vi "OCR Get Names.vi"(7 "error in":errorcluster, 10 "SS Path":path=path "c:/PokerSS/SS.png") -> (0 "error out":errorcluster, 3 "Player Names":string[](array[string]))   [LabVIEW 2015]
uses:
  <vilib>/vision/NI_Vision_Development_Module.lvlib
panel:
  out "Image Out":T1(plugin-control)
  out "String ( Player10 OCR/OCV 4)":string
  out "String (Player9 OCR/OCV 4)":string
  out "String (Player8 OCR/OCV 4)":string
  out "String (Player7 OCR/OCV 4)":string
  out "String (Playe6 OCR/OCV 4)":string
  out "String (Player5 OCR/OCV 4)":string
  out "String (Player4 OCR/OCV 4)":string
  out "String (Player3 OCR/OCV 4)":string
  out "String (Player2 OCR/OCV 4)":string
  out "String (Player1 OCR/OCV 4)":string
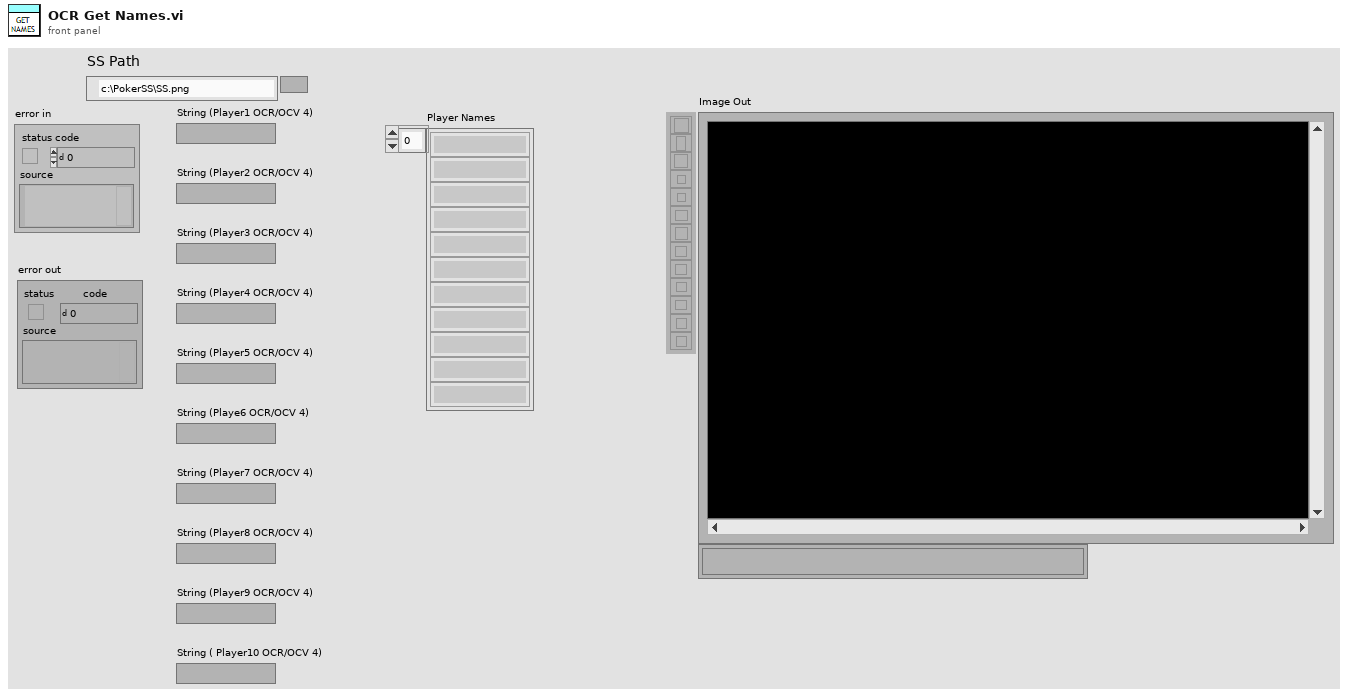
[diagram p1: front panel]
types:
  T1 = typedef "IMAQ Image.ctl" = refnum<image>
  T2 = cluster{"Threshold Data":cluster{"Method":enum16{"Fixed Range", "Uniform", "Linear", "Non Linear", "Local", "Color"}, "Looking for":u32, "Color Mode":u32, "Kernel Size":cluster{"Width":i32, "Height":i32}, "Ranges":cluster{"Min":i32, "Max":i32}[]}, "Reject Border":bool, "Number Of Erosions":i32, "Size & Spacing":cluster{"Segment Algorithm":u16, "Min Bounding Rect Width":i32, "Max Bounding Rect Width":i32, "Min Bounding Rect Height":i32, "Max Bounding Rect Height":i32, "Min Character Size":i32, "Max Character Size":i32, "Min Char Spacing":i32, "Max Horiz Element Spacing":i32, "Max Vert Element Spacing":i32, "Max Space Distance":i32}, "Read Options":cluster{"Read Strategy":i32, "Read Resolution":i32, "Scale Dependant":bool, "Aspect Ratio":i32, "Acceptance Level":i32, "Substitution Character":string, "MultiLine":bool}, "Valid Characters":cluster{"Pre-defined characters":i32, "User-defined characters":string}[], "Use Text Pattern":bool, "Orientation":u32, "# Lines Expected":u32, "Number of Blocks":i32}
  T3 = cluster{"Global Rectangle":i32[], "Contours":cluster{"ID":enum32{"External", "Internal"}, "Type":u32, "Coordinates":i32[]}[]}
  T4 = typedef "Image Type" = u32
  T5 = typedef "IMAQ OCR Session.ctl" = refnum<k1>
diagram:
  w25 = u32 0 items=["Grayscale", "Binary", "Gradient", "Rainbow", "Temperature", "User Defined", "Binary 16 Bit", "Gradient 16 Bit", "Rainbow 16 Bit", "Temperature 16 Bit", "User Defined 16 Bit"] ("Palette Type")
  w34 = T2 {"Threshold Data"={"Method"=enum."Linear", "Looking for"=1, "Color Mode"=0, "Kernel Size"={"Width"=32, "Height"=32}, "Ranges"=[{"Min"=1, "Max"=255}]}, "Reject Border"=TRUE, "Number Of Erosions"=0, "Size & Spacing"={"Segment Algorithm"=0, "Min Bounding Rect Width"=2, "Max Bounding Rect Width"=7, "Min Bounding Rect Height"=2, "Max Bounding Rect Height"=65536, "Min Character Size"=4, "Max Character Size"=5555, "Min Char Spacing"=1, "Max Horiz Element Spacing"=1, "Max Vert Element Spacing"=0, "Max Space Distance"=65536}, "Read Options"={"Read Strategy"=1, "Read Resolution"=2, "Scale Dependant"=FALSE, "Aspect Ratio"=400, "Acceptance Level"=700, "Substitution Character"="?", "MultiLine"=FALSE}, "Valid Characters"=[], "Use Text Pattern"=FALSE, "Orientation"=0, "# Lines Expected"=0, "Number of Blocks"=4}  # Parameters
  w35 = T3 {"Global Rectangle"=[718, 479, 831, 496], "Contours"=[{"ID"=enum."External", "Type"=3, "Coordinates"=[718, 479, 831, 496]}]}  # ROI Descriptor
  w43 = T2 {"Threshold Data"={"Method"=enum."Linear", "Looking for"=1, "Color Mode"=0, "Kernel Size"={"Width"=32, "Height"=32}, "Ranges"=[{"Min"=1, "Max"=255}]}, "Reject Border"=TRUE, "Number Of Erosions"=0, "Size & Spacing"={"Segment Algorithm"=0, "Min Bounding Rect Width"=2, "Max Bounding Rect Width"=7, "Min Bounding Rect Height"=2, "Max Bounding Rect Height"=65536, "Min Character Size"=4, "Max Character Size"=5555, "Min Char Spacing"=1, "Max Horiz Element Spacing"=1, "Max Vert Element Spacing"=0, "Max Space Distance"=65536}, "Read Options"={"Read Strategy"=1, "Read Resolution"=2, "Scale Dependant"=FALSE, "Aspect Ratio"=400, "Acceptance Level"=700, "Substitution Character"="?", "MultiLine"=FALSE}, "Valid Characters"=[], "Use Text Pattern"=FALSE, "Orientation"=0, "# Lines Expected"=0, "Number of Blocks"=4}  # Parameters
  w44 = T3 {"Global Rectangle"=[523, 517, 648, 536], "Contours"=[{"ID"=enum."External", "Type"=3, "Coordinates"=[523, 517, 648, 536]}]}  # ROI Descriptor
  w52 = T2 {"Threshold Data"={"Method"=enum."Linear", "Looking for"=1, "Color Mode"=0, "Kernel Size"={"Width"=32, "Height"=32}, "Ranges"=[{"Min"=1, "Max"=255}]}, "Reject Border"=TRUE, "Number Of Erosions"=0, "Size & Spacing"={"Segment Algorithm"=0, "Min Bounding Rect Width"=2, "Max Bounding Rect Width"=7, "Min Bounding Rect Height"=2, "Max Bounding Rect Height"=65536, "Min Character Size"=4, "Max Character Size"=5555, "Min Char Spacing"=1, "Max Horiz Element Spacing"=1, "Max Vert Element Spacing"=0, "Max Space Distance"=65536}, "Read Options"={"Read Strategy"=1, "Read Resolution"=2, "Scale Dependant"=FALSE, "Aspect Ratio"=400, "Acceptance Level"=700, "Substitution Character"="?", "MultiLine"=FALSE}, "Valid Characters"=[], "Use Text Pattern"=FALSE, "Orientation"=0, "# Lines Expected"=0, "Number of Blocks"=4}  # Parameters
  w53 = T3 {"Global Rectangle"=[389, 674, 500, 690], "Contours"=[{"ID"=enum."External", "Type"=3, "Coordinates"=[389, 674, 500, 690]}]}  # ROI Descriptor
  w61 = T2 {"Threshold Data"={"Method"=enum."Linear", "Looking for"=1, "Color Mode"=0, "Kernel Size"={"Width"=32, "Height"=32}, "Ranges"=[{"Min"=1, "Max"=255}]}, "Reject Border"=TRUE, "Number Of Erosions"=0, "Size & Spacing"={"Segment Algorithm"=0, "Min Bounding Rect Width"=2, "Max Bounding Rect Width"=7, "Min Bounding Rect Height"=2, "Max Bounding Rect Height"=65536, "Min Character Size"=4, "Max Character Size"=5555, "Min Char Spacing"=1, "Max Horiz Element Spacing"=1, "Max Vert Element Spacing"=0, "Max Space Distance"=65536}, "Read Options"={"Read Strategy"=1, "Read Resolution"=2, "Scale Dependant"=FALSE, "Aspect Ratio"=400, "Acceptance Level"=700, "Substitution Character"="?", "MultiLine"=FALSE}, "Valid Characters"=[], "Use Text Pattern"=FALSE, "Orientation"=0, "# Lines Expected"=0, "Number of Blocks"=4}  # Parameters
  w62 = T3 {"Global Rectangle"=[539, 820, 663, 837], "Contours"=[{"ID"=enum."External", "Type"=3, "Coordinates"=[539, 820, 663, 837]}]}  # ROI Descriptor
  w70 = T2 {"Threshold Data"={"Method"=enum."Linear", "Looking for"=1, "Color Mode"=0, "Kernel Size"={"Width"=32, "Height"=32}, "Ranges"=[{"Min"=1, "Max"=255}]}, "Reject Border"=TRUE, "Number Of Erosions"=0, "Size & Spacing"={"Segment Algorithm"=0, "Min Bounding Rect Width"=2, "Max Bounding Rect Width"=7, "Min Bounding Rect Height"=2, "Max Bounding Rect Height"=65536, "Min Character Size"=4, "Max Character Size"=5555, "Min Char Spacing"=1, "Max Horiz Element Spacing"=1, "Max Vert Element Spacing"=0, "Max Space Distance"=65536}, "Read Options"={"Read Strategy"=1, "Read Resolution"=2, "Scale Dependant"=FALSE, "Aspect Ratio"=400, "Acceptance Level"=700, "Substitution Character"="?", "MultiLine"=FALSE}, "Valid Characters"=[], "Use Text Pattern"=FALSE, "Orientation"=0, "# Lines Expected"=0, "Number of Blocks"=4}  # Parameters
  w71 = T3 {"Global Rectangle"=[758, 853, 874, 871], "Contours"=[{"ID"=enum."External", "Type"=3, "Coordinates"=[758, 853, 874, 871]}]}  # ROI Descriptor
  w79 = T2 {"Threshold Data"={"Method"=enum."Linear", "Looking for"=1, "Color Mode"=0, "Kernel Size"={"Width"=32, "Height"=32}, "Ranges"=[{"Min"=1, "Max"=255}]}, "Reject Border"=TRUE, "Number Of Erosions"=0, "Size & Spacing"={"Segment Algorithm"=0, "Min Bounding Rect Width"=2, "Max Bounding Rect Width"=7, "Min Bounding Rect Height"=2, "Max Bounding Rect Height"=65536, "Min Character Size"=4, "Max Character Size"=5555, "Min Char Spacing"=1, "Max Horiz Element Spacing"=1, "Max Vert Element Spacing"=0, "Max Space Distance"=65536}, "Read Options"={"Read Strategy"=1, "Read Resolution"=2, "Scale Dependant"=FALSE, "Aspect Ratio"=400, "Acceptance Level"=700, "Substitution Character"="?", "MultiLine"=FALSE}, "Valid Characters"=[], "Use Text Pattern"=FALSE, "Orientation"=0, "# Lines Expected"=0, "Number of Blocks"=4}  # Parameters
  w80 = T3 {"Global Rectangle"=[1028, 852, 1145, 868], "Contours"=[{"ID"=enum."External", "Type"=3, "Coordinates"=[1028, 852, 1145, 868]}]}  # ROI Descriptor
  w88 = T2 {"Threshold Data"={"Method"=enum."Linear", "Looking for"=1, "Color Mode"=0, "Kernel Size"={"Width"=32, "Height"=32}, "Ranges"=[{"Min"=1, "Max"=255}]}, "Reject Border"=TRUE, "Number Of Erosions"=0, "Size & Spacing"={"Segment Algorithm"=0, "Min Bounding Rect Width"=2, "Max Bounding Rect Width"=7, "Min Bounding Rect Height"=2, "Max Bounding Rect Height"=65536, "Min Character Size"=4, "Max Character Size"=5555, "Min Char Spacing"=1, "Max Horiz Element Spacing"=1, "Max Vert Element Spacing"=0, "Max Space Distance"=65536}, "Read Options"={"Read Strategy"=1, "Read Resolution"=2, "Scale Dependant"=FALSE, "Aspect Ratio"=400, "Acceptance Level"=700, "Substitution Character"="?", "MultiLine"=FALSE}, "Valid Characters"=[], "Use Text Pattern"=FALSE, "Orientation"=0, "# Lines Expected"=0, "Number of Blocks"=4}  # Parameters
  w89 = T3 {"Global Rectangle"=[1255, 819, 1378, 838], "Contours"=[{"ID"=enum."External", "Type"=3, "Coordinates"=[1255, 819, 1378, 838]}]}  # ROI Descriptor
  w97 = T2 {"Threshold Data"={"Method"=enum."Linear", "Looking for"=1, "Color Mode"=0, "Kernel Size"={"Width"=32, "Height"=32}, "Ranges"=[{"Min"=1, "Max"=255}]}, "Reject Border"=TRUE, "Number Of Erosions"=0, "Size & Spacing"={"Segment Algorithm"=0, "Min Bounding Rect Width"=2, "Max Bounding Rect Width"=7, "Min Bounding Rect Height"=2, "Max Bounding Rect Height"=65536, "Min Character Size"=4, "Max Character Size"=5555, "Min Char Spacing"=1, "Max Horiz Element Spacing"=1, "Max Vert Element Spacing"=0, "Max Space Distance"=65536}, "Read Options"={"Read Strategy"=1, "Read Resolution"=2, "Scale Dependant"=FALSE, "Aspect Ratio"=400, "Acceptance Level"=700, "Substitution Character"="?", "MultiLine"=FALSE}, "Valid Characters"=[], "Use Text Pattern"=FALSE, "Orientation"=0, "# Lines Expected"=0, "Number of Blocks"=4}  # Parameters
  w98 = T3 {"Global Rectangle"=[1387, 681, 1506, 696], "Contours"=[{"ID"=enum."External", "Type"=3, "Coordinates"=[1387, 681, 1506, 696]}]}  # ROI Descriptor
  w106 = T2 {"Threshold Data"={"Method"=enum."Linear", "Looking for"=1, "Color Mode"=0, "Kernel Size"={"Width"=32, "Height"=32}, "Ranges"=[{"Min"=1, "Max"=255}]}, "Reject Border"=TRUE, "Number Of Erosions"=0, "Size & Spacing"={"Segment Algorithm"=0, "Min Bounding Rect Width"=2, "Max Bounding Rect Width"=7, "Min Bounding Rect Height"=2, "Max Bounding Rect Height"=65536, "Min Character Size"=4, "Max Character Size"=5555, "Min Char Spacing"=1, "Max Horiz Element Spacing"=1, "Max Vert Element Spacing"=0, "Max Space Distance"=65536}, "Read Options"={"Read Strategy"=1, "Read Resolution"=2, "Scale Dependant"=FALSE, "Aspect Ratio"=400, "Acceptance Level"=700, "Substitution Character"="?", "MultiLine"=FALSE}, "Valid Characters"=[], "Use Text Pattern"=FALSE, "Orientation"=0, "# Lines Expected"=0, "Number of Blocks"=4}  # Parameters
  w107 = T3 {"Global Rectangle"=[1248, 519, 1366, 535], "Contours"=[{"ID"=enum."External", "Type"=3, "Coordinates"=[1248, 519, 1366, 535]}]}  # ROI Descriptor
  w115 = T2 {"Threshold Data"={"Method"=enum."Linear", "Looking for"=1, "Color Mode"=0, "Kernel Size"={"Width"=32, "Height"=32}, "Ranges"=[{"Min"=1, "Max"=255}]}, "Reject Border"=TRUE, "Number Of Erosions"=0, "Size & Spacing"={"Segment Algorithm"=0, "Min Bounding Rect Width"=2, "Max Bounding Rect Width"=7, "Min Bounding Rect Height"=2, "Max Bounding Rect Height"=65536, "Min Character Size"=4, "Max Character Size"=5555, "Min Char Spacing"=1, "Max Horiz Element Spacing"=1, "Max Vert Element Spacing"=0, "Max Space Distance"=65536}, "Read Options"={"Read Strategy"=1, "Read Resolution"=2, "Scale Dependant"=FALSE, "Aspect Ratio"=400, "Acceptance Level"=700, "Substitution Character"="?", "MultiLine"=FALSE}, "Valid Characters"=[], "Use Text Pattern"=FALSE, "Orientation"=0, "# Lines Expected"=0, "Number of Blocks"=4}  # Parameters
  w116 = T3 {"Global Rectangle"=[1075, 479, 1162, 494], "Contours"=[{"ID"=enum."External", "Type"=3, "Coordinates"=[1075, 479, 1162, 494]}]}  # ROI Descriptor
  w120 = 1 items=["Red", "Green", "Blue", "Hue", "Saturation", "Luminance", "Value", "Intensity"] ("Color Plane")
  w121 = T4 4 items=["Grayscale (U8)", "Grayscale (I16)", "Grayscale (SGL)", "Complex (CSG)", "RGB (U32)", "HSL (U32)", "RGB (U64)", "Grayscale (U16)"] ("Image Type")
  n1 = Call Chain() -> (call chain=w123:string[])
  n2 = Index Array(array=w123) -> (element=w122:string)  [unwired: 1 in]
  n3 = call "IMAQ Create"("Image Name"=w122, "Image Type"=w121, "error in (no error)"="error in") -> ("New Image"=w126:T1, "error out"=w125:errorcluster)  [unwired: 1 in, 1 out]
  n4 = call "IMAQ ReadFile"("File Path"="SS Path", "error in (no error)"=w125, "Image"=w126) -> ("error out"=w127:errorcluster, "Image Out"=w119:T1)  [unwired: 2 in, 5 out]
  n5 = call "IMAQ ExtractSingleColorPlane"("Color Plane"=w120, "error in (no error)"=w127, "Image Src"=w119) -> ("error out"=w118:errorcluster, "Image Dst Out"=w26:T1)  [unwired: 1 in, 6 out]
  "Image Out" <- w26
  n6 = while "Create an OCR session and read the character set file.\nSet paramaters from Vision Assistant Step." {
    shift-right: [w132] -> w113
    shift-left: _ -> [w131]
    tunnel: w118 -> [w134]
    tunnel: w115 -> [w130]
    tunnel: path "C:/Users/Bob Dabalina/Documents/Labview/Poker Hand2/Viewsonic1.abc" ("File Path") -> [w129]
    tunnel: [w128] -> w114
    stop <- FALSE continue-if-true
    n7 = First Call?() -> (First Call?: T/F=w133:bool)
    n8 = case shown="True" w133 {
      tunnel: w129 -> [_ w141]
      tunnel: w134 -> [w136 w145]
      tunnel: [w137 w143] -> w132
      tunnel: [w136 w142] -> w128
      tunnel: w130 -> [_ w138]
      tunnel: w131 -> [w137 _]
      frame False {
      }
      frame True {
        w146 = 0 items=["Read All", "Read Character Set Only", "Read Properties Only"] ("Read Options")
        n9 = call <vilib>:"IVA Get Alternate Path.vi"("Path In"=w141) -> ("Path Out"=w140:path)  [unwired: 10 out]
        n10 = call "IMAQ OCR Create Session"("error in (no error)"=w145) -> ("error out"=w147:errorcluster, "IMAQ OCR Session"=w148:T5)  [unwired: 9 out]
        n11 = call "IMAQ OCR Read Character Set File"("File Path"=w140, "error in (no error)"=w147, "Read Options"=w146, "IMAQ OCR Session"=w148) -> ("error out"=w144:errorcluster, "IMAQ OCR Session (dup)"=w139:T5)  [unwired: 1 in, 5 out]
        n12 = call <vilib>:"IVA OCR - Set Parameters 2.vi"("error in (no error)"=w144, "Parameters"=w138, "IMAQ OCR Session"=w139) -> ("error out"=w142:errorcluster, "IMAQ OCR Session Out"=w143:T5)  [unwired: 7 in]
      }
    }
  }
  n13 = Unbundle By Name(w115) -> ("# Lines Expected"=w111:u32, "Orientation"=w112:u32)
  n14 = Initialize Array "Initialize Array"("") -> (w23:string[])  [unwired: 1 in]
  n15 = call "IMAQ OCR Read Text 4"("IMAQ OCR Session"=w113, "ROI Descriptor"=w116, "Image"=w26, "Number of Lines Requested"=w111, "error in (no error)"=w114, "Orientation"=w112) -> ("Read String"=w21:string, "error out"=w110:errorcluster)  [unwired: 8 out]
  "String (Player1 OCR/OCV 4)" <- w21
  n16 = Insert Into Array "Insert Into Array"(array=w23, index=0, new element=w21) -> (w20:string[])
  n17 = call <vilib>:"IVA Clear Coordsys Errors.vi"("error in (no error)"=w110) -> ("error out"=w109:errorcluster)  [unwired: 10 in]
  n18 = while "Create an OCR session and read the character set file.\nSet paramaters from Vision Assistant Step." {
    shift-right: [w153] -> w104
    shift-left: _ -> [w152]
    tunnel: w109 -> [w155]
    tunnel: w106 -> [w151]
    tunnel: path "C:/Users/Bob Dabalina/Documents/Labview/Poker Hand2/Viewsonic1.abc" ("File Path") -> [w150]
    tunnel: [w149] -> w105
    stop <- FALSE continue-if-true
    n19 = First Call?() -> (First Call?: T/F=w154:bool)
    n20 = case shown="True" w154 {
      tunnel: w150 -> [_ w162]
      tunnel: w155 -> [w157 w166]
      tunnel: [w158 w164] -> w153
      tunnel: [w157 w163] -> w149
      tunnel: w151 -> [_ w159]
      tunnel: w152 -> [w158 _]
      frame False {
      }
      frame True {
        w167 = 0 items=["Read All", "Read Character Set Only", "Read Properties Only"] ("Read Options")
        n21 = call <vilib>:"IVA Get Alternate Path.vi"("Path In"=w162) -> ("Path Out"=w161:path)  [unwired: 10 out]
        n22 = call "IMAQ OCR Create Session"("error in (no error)"=w166) -> ("error out"=w168:errorcluster, "IMAQ OCR Session"=w169:T5)  [unwired: 9 out]
        n23 = call "IMAQ OCR Read Character Set File"("File Path"=w161, "error in (no error)"=w168, "Read Options"=w167, "IMAQ OCR Session"=w169) -> ("error out"=w165:errorcluster, "IMAQ OCR Session (dup)"=w160:T5)  [unwired: 1 in, 5 out]
        n24 = call <vilib>:"IVA OCR - Set Parameters 2.vi"("error in (no error)"=w165, "Parameters"=w159, "IMAQ OCR Session"=w160) -> ("error out"=w163:errorcluster, "IMAQ OCR Session Out"=w164:T5)  [unwired: 7 in]
      }
    }
  }
  n25 = Unbundle By Name(w106) -> ("# Lines Expected"=w102:u32, "Orientation"=w103:u32)
  n26 = call "IMAQ OCR Read Text 4"("IMAQ OCR Session"=w104, "ROI Descriptor"=w107, "Image"=w26, "Number of Lines Requested"=w102, "error in (no error)"=w105, "Orientation"=w103) -> ("Read String"=w19:string, "error out"=w101:errorcluster)  [unwired: 8 out]
  "String (Player2 OCR/OCV 4)" <- w19
  n27 = Build Array (concatenate)(w20, w19) -> (w18:string[])
  n28 = call <vilib>:"IVA Clear Coordsys Errors.vi"("error in (no error)"=w101) -> ("error out"=w100:errorcluster)  [unwired: 10 in]
  n29 = while "Create an OCR session and read the character set file.\nSet paramaters from Vision Assistant Step." {
    shift-right: [w174] -> w95
    shift-left: _ -> [w173]
    tunnel: w100 -> [w176]
    tunnel: w97 -> [w172]
    tunnel: path "C:/Users/Bob Dabalina/Documents/Labview/Poker Hand2/Viewsonic1.abc" ("File Path") -> [w171]
    tunnel: [w170] -> w96
    stop <- FALSE continue-if-true
    n30 = First Call?() -> (First Call?: T/F=w175:bool)
    n31 = case shown="True" w175 {
      tunnel: w171 -> [_ w183]
      tunnel: w176 -> [w178 w187]
      tunnel: [w179 w185] -> w174
      tunnel: [w178 w184] -> w170
      tunnel: w172 -> [_ w180]
      tunnel: w173 -> [w179 _]
      frame False {
      }
      frame True {
        w188 = 0 items=["Read All", "Read Character Set Only", "Read Properties Only"] ("Read Options")
        n32 = call <vilib>:"IVA Get Alternate Path.vi"("Path In"=w183) -> ("Path Out"=w182:path)  [unwired: 10 out]
        n33 = call "IMAQ OCR Create Session"("error in (no error)"=w187) -> ("error out"=w189:errorcluster, "IMAQ OCR Session"=w190:T5)  [unwired: 9 out]
        n34 = call "IMAQ OCR Read Character Set File"("File Path"=w182, "error in (no error)"=w189, "Read Options"=w188, "IMAQ OCR Session"=w190) -> ("error out"=w186:errorcluster, "IMAQ OCR Session (dup)"=w181:T5)  [unwired: 1 in, 5 out]
        n35 = call <vilib>:"IVA OCR - Set Parameters 2.vi"("error in (no error)"=w186, "Parameters"=w180, "IMAQ OCR Session"=w181) -> ("error out"=w184:errorcluster, "IMAQ OCR Session Out"=w185:T5)  [unwired: 7 in]
      }
    }
  }
  n36 = Unbundle By Name(w97) -> ("# Lines Expected"=w93:u32, "Orientation"=w94:u32)
  n37 = call "IMAQ OCR Read Text 4"("IMAQ OCR Session"=w95, "ROI Descriptor"=w98, "Image"=w26, "Number of Lines Requested"=w93, "error in (no error)"=w96, "Orientation"=w94) -> ("Read String"=w17:string, "error out"=w92:errorcluster)  [unwired: 8 out]
  "String (Player3 OCR/OCV 4)" <- w17
  n38 = Build Array (concatenate)(w18, w17) -> (w16:string[])
  n39 = call <vilib>:"IVA Clear Coordsys Errors.vi"("error in (no error)"=w92) -> ("error out"=w91:errorcluster)  [unwired: 10 in]
  n40 = while "Create an OCR session and read the character set file.\nSet paramaters from Vision Assistant Step." {
    shift-right: [w195] -> w86
    shift-left: _ -> [w194]
    tunnel: w91 -> [w197]
    tunnel: w88 -> [w193]
    tunnel: path "C:/Users/Bob Dabalina/Documents/Labview/Poker Hand2/Viewsonic1.abc" ("File Path") -> [w192]
    tunnel: [w191] -> w87
    stop <- FALSE continue-if-true
    n41 = First Call?() -> (First Call?: T/F=w196:bool)
    n42 = case shown="True" w196 {
      tunnel: w192 -> [_ w204]
      tunnel: w197 -> [w199 w208]
      tunnel: [w200 w206] -> w195
      tunnel: [w199 w205] -> w191
      tunnel: w193 -> [_ w201]
      tunnel: w194 -> [w200 _]
      frame False {
      }
      frame True {
        w209 = 0 items=["Read All", "Read Character Set Only", "Read Properties Only"] ("Read Options")
        n43 = call <vilib>:"IVA Get Alternate Path.vi"("Path In"=w204) -> ("Path Out"=w203:path)  [unwired: 10 out]
        n44 = call "IMAQ OCR Create Session"("error in (no error)"=w208) -> ("error out"=w210:errorcluster, "IMAQ OCR Session"=w211:T5)  [unwired: 9 out]
        n45 = call "IMAQ OCR Read Character Set File"("File Path"=w203, "error in (no error)"=w210, "Read Options"=w209, "IMAQ OCR Session"=w211) -> ("error out"=w207:errorcluster, "IMAQ OCR Session (dup)"=w202:T5)  [unwired: 1 in, 5 out]
        n46 = call <vilib>:"IVA OCR - Set Parameters 2.vi"("error in (no error)"=w207, "Parameters"=w201, "IMAQ OCR Session"=w202) -> ("error out"=w205:errorcluster, "IMAQ OCR Session Out"=w206:T5)  [unwired: 7 in]
      }
    }
  }
  n47 = Unbundle By Name(w88) -> ("# Lines Expected"=w84:u32, "Orientation"=w85:u32)
  n48 = call "IMAQ OCR Read Text 4"("IMAQ OCR Session"=w86, "ROI Descriptor"=w89, "Image"=w26, "Number of Lines Requested"=w84, "error in (no error)"=w87, "Orientation"=w85) -> ("Read String"=w15:string, "error out"=w83:errorcluster)  [unwired: 8 out]
  "String (Player4 OCR/OCV 4)" <- w15
  n49 = Build Array (concatenate)(w16, w15) -> (w14:string[])
  n50 = call <vilib>:"IVA Clear Coordsys Errors.vi"("error in (no error)"=w83) -> ("error out"=w82:errorcluster)  [unwired: 10 in]
  n51 = while "Create an OCR session and read the character set file.\nSet paramaters from Vision Assistant Step." {
    shift-right: [w216] -> w77
    shift-left: _ -> [w215]
    tunnel: w82 -> [w218]
    tunnel: w79 -> [w214]
    tunnel: path "C:/Users/Bob Dabalina/Documents/Labview/Poker Hand2/Viewsonic1.abc" ("File Path") -> [w213]
    tunnel: [w212] -> w78
    stop <- FALSE continue-if-true
    n52 = First Call?() -> (First Call?: T/F=w217:bool)
    n53 = case shown="True" w217 {
      tunnel: w213 -> [_ w225]
      tunnel: w218 -> [w220 w229]
      tunnel: [w221 w227] -> w216
      tunnel: [w220 w226] -> w212
      tunnel: w214 -> [_ w222]
      tunnel: w215 -> [w221 _]
      frame False {
      }
      frame True {
        w230 = 0 items=["Read All", "Read Character Set Only", "Read Properties Only"] ("Read Options")
        n54 = call <vilib>:"IVA Get Alternate Path.vi"("Path In"=w225) -> ("Path Out"=w224:path)  [unwired: 10 out]
        n55 = call "IMAQ OCR Create Session"("error in (no error)"=w229) -> ("error out"=w231:errorcluster, "IMAQ OCR Session"=w232:T5)  [unwired: 9 out]
        n56 = call "IMAQ OCR Read Character Set File"("File Path"=w224, "error in (no error)"=w231, "Read Options"=w230, "IMAQ OCR Session"=w232) -> ("error out"=w228:errorcluster, "IMAQ OCR Session (dup)"=w223:T5)  [unwired: 1 in, 5 out]
        n57 = call <vilib>:"IVA OCR - Set Parameters 2.vi"("error in (no error)"=w228, "Parameters"=w222, "IMAQ OCR Session"=w223) -> ("error out"=w226:errorcluster, "IMAQ OCR Session Out"=w227:T5)  [unwired: 7 in]
      }
    }
  }
  n58 = Unbundle By Name(w79) -> ("# Lines Expected"=w75:u32, "Orientation"=w76:u32)
  n59 = call "IMAQ OCR Read Text 4"("IMAQ OCR Session"=w77, "ROI Descriptor"=w80, "Image"=w26, "Number of Lines Requested"=w75, "error in (no error)"=w78, "Orientation"=w76) -> ("Read String"=w13:string, "error out"=w74:errorcluster)  [unwired: 8 out]
  "String (Player5 OCR/OCV 4)" <- w13
  n60 = Build Array (concatenate)(w14, w13) -> (w12:string[])
  n61 = call <vilib>:"IVA Clear Coordsys Errors.vi"("error in (no error)"=w74) -> ("error out"=w73:errorcluster)  [unwired: 10 in]
  n62 = while "Create an OCR session and read the character set file.\nSet paramaters from Vision Assistant Step." {
    shift-right: [w237] -> w68
    shift-left: _ -> [w236]
    tunnel: w73 -> [w239]
    tunnel: w70 -> [w235]
    tunnel: path "C:/Users/Bob Dabalina/Documents/Labview/Poker Hand2/Viewsonic1.abc" ("File Path") -> [w234]
    tunnel: [w233] -> w69
    stop <- FALSE continue-if-true
    n63 = First Call?() -> (First Call?: T/F=w238:bool)
    n64 = case shown="True" w238 {
      tunnel: w234 -> [_ w246]
      tunnel: w239 -> [w241 w250]
      tunnel: [w242 w248] -> w237
      tunnel: [w241 w247] -> w233
      tunnel: w235 -> [_ w243]
      tunnel: w236 -> [w242 _]
      frame False {
      }
      frame True {
        w251 = 0 items=["Read All", "Read Character Set Only", "Read Properties Only"] ("Read Options")
        n65 = call <vilib>:"IVA Get Alternate Path.vi"("Path In"=w246) -> ("Path Out"=w245:path)  [unwired: 10 out]
        n66 = call "IMAQ OCR Create Session"("error in (no error)"=w250) -> ("error out"=w252:errorcluster, "IMAQ OCR Session"=w253:T5)  [unwired: 9 out]
        n67 = call "IMAQ OCR Read Character Set File"("File Path"=w245, "error in (no error)"=w252, "Read Options"=w251, "IMAQ OCR Session"=w253) -> ("error out"=w249:errorcluster, "IMAQ OCR Session (dup)"=w244:T5)  [unwired: 1 in, 5 out]
        n68 = call <vilib>:"IVA OCR - Set Parameters 2.vi"("error in (no error)"=w249, "Parameters"=w243, "IMAQ OCR Session"=w244) -> ("error out"=w247:errorcluster, "IMAQ OCR Session Out"=w248:T5)  [unwired: 7 in]
      }
    }
  }
  n69 = Unbundle By Name(w70) -> ("# Lines Expected"=w66:u32, "Orientation"=w67:u32)
  n70 = call "IMAQ OCR Read Text 4"("IMAQ OCR Session"=w68, "ROI Descriptor"=w71, "Image"=w26, "Number of Lines Requested"=w66, "error in (no error)"=w69, "Orientation"=w67) -> ("Read String"=w11:string, "error out"=w65:errorcluster)  [unwired: 8 out]
  "String (Playe6 OCR/OCV 4)" <- w11
  n71 = Build Array (concatenate)(w12, w11) -> (w10:string[])
  n72 = call <vilib>:"IVA Clear Coordsys Errors.vi"("error in (no error)"=w65) -> ("error out"=w64:errorcluster)  [unwired: 10 in]
  n73 = while "Create an OCR session and read the character set file.\nSet paramaters from Vision Assistant Step." {
    shift-right: [w258] -> w59
    shift-left: _ -> [w257]
    tunnel: w64 -> [w260]
    tunnel: w61 -> [w256]
    tunnel: path "C:/Users/Bob Dabalina/Documents/Labview/Poker Hand2/Viewsonic1.abc" ("File Path") -> [w255]
    tunnel: [w254] -> w60
    stop <- FALSE continue-if-true
    n74 = First Call?() -> (First Call?: T/F=w259:bool)
    n75 = case shown="True" w259 {
      tunnel: w255 -> [_ w267]
      tunnel: w260 -> [w262 w271]
      tunnel: [w263 w269] -> w258
      tunnel: [w262 w268] -> w254
      tunnel: w256 -> [_ w264]
      tunnel: w257 -> [w263 _]
      frame False {
      }
      frame True {
        w272 = 0 items=["Read All", "Read Character Set Only", "Read Properties Only"] ("Read Options")
        n76 = call <vilib>:"IVA Get Alternate Path.vi"("Path In"=w267) -> ("Path Out"=w266:path)  [unwired: 10 out]
        n77 = call "IMAQ OCR Create Session"("error in (no error)"=w271) -> ("error out"=w273:errorcluster, "IMAQ OCR Session"=w274:T5)  [unwired: 9 out]
        n78 = call "IMAQ OCR Read Character Set File"("File Path"=w266, "error in (no error)"=w273, "Read Options"=w272, "IMAQ OCR Session"=w274) -> ("error out"=w270:errorcluster, "IMAQ OCR Session (dup)"=w265:T5)  [unwired: 1 in, 5 out]
        n79 = call <vilib>:"IVA OCR - Set Parameters 2.vi"("error in (no error)"=w270, "Parameters"=w264, "IMAQ OCR Session"=w265) -> ("error out"=w268:errorcluster, "IMAQ OCR Session Out"=w269:T5)  [unwired: 7 in]
      }
    }
  }
  n80 = Unbundle By Name(w61) -> ("# Lines Expected"=w57:u32, "Orientation"=w58:u32)
  n81 = call "IMAQ OCR Read Text 4"("IMAQ OCR Session"=w59, "ROI Descriptor"=w62, "Image"=w26, "Number of Lines Requested"=w57, "error in (no error)"=w60, "Orientation"=w58) -> ("Read String"=w9:string, "error out"=w56:errorcluster)  [unwired: 8 out]
  "String (Player7 OCR/OCV 4)" <- w9
  n82 = Build Array (concatenate)(w10, w9) -> (w8:string[])
  n83 = call <vilib>:"IVA Clear Coordsys Errors.vi"("error in (no error)"=w56) -> ("error out"=w55:errorcluster)  [unwired: 10 in]
  n84 = while "Create an OCR session and read the character set file.\nSet paramaters from Vision Assistant Step." {
    shift-right: [w279] -> w50
    shift-left: _ -> [w278]
    tunnel: w55 -> [w281]
    tunnel: w52 -> [w277]
    tunnel: path "C:/Users/Bob Dabalina/Documents/Labview/Poker Hand2/Viewsonic1.abc" ("File Path") -> [w276]
    tunnel: [w275] -> w51
    stop <- FALSE continue-if-true
    n85 = First Call?() -> (First Call?: T/F=w280:bool)
    n86 = case shown="True" w280 {
      tunnel: w276 -> [_ w288]
      tunnel: w281 -> [w283 w292]
      tunnel: [w284 w290] -> w279
      tunnel: [w283 w289] -> w275
      tunnel: w277 -> [_ w285]
      tunnel: w278 -> [w284 _]
      frame False {
      }
      frame True {
        w293 = 0 items=["Read All", "Read Character Set Only", "Read Properties Only"] ("Read Options")
        n87 = call <vilib>:"IVA Get Alternate Path.vi"("Path In"=w288) -> ("Path Out"=w287:path)  [unwired: 10 out]
        n88 = call "IMAQ OCR Create Session"("error in (no error)"=w292) -> ("error out"=w294:errorcluster, "IMAQ OCR Session"=w295:T5)  [unwired: 9 out]
        n89 = call "IMAQ OCR Read Character Set File"("File Path"=w287, "error in (no error)"=w294, "Read Options"=w293, "IMAQ OCR Session"=w295) -> ("error out"=w291:errorcluster, "IMAQ OCR Session (dup)"=w286:T5)  [unwired: 1 in, 5 out]
        n90 = call <vilib>:"IVA OCR - Set Parameters 2.vi"("error in (no error)"=w291, "Parameters"=w285, "IMAQ OCR Session"=w286) -> ("error out"=w289:errorcluster, "IMAQ OCR Session Out"=w290:T5)  [unwired: 7 in]
      }
    }
  }
  n91 = Unbundle By Name(w52) -> ("# Lines Expected"=w48:u32, "Orientation"=w49:u32)
  n92 = call "IMAQ OCR Read Text 4"("IMAQ OCR Session"=w50, "ROI Descriptor"=w53, "Image"=w26, "Number of Lines Requested"=w48, "error in (no error)"=w51, "Orientation"=w49) -> ("Read String"=w7:string, "error out"=w47:errorcluster)  [unwired: 8 out]
  "String (Player8 OCR/OCV 4)" <- w7
  n93 = Build Array (concatenate)(w8, w7) -> (w6:string[])
  n94 = call <vilib>:"IVA Clear Coordsys Errors.vi"("error in (no error)"=w47) -> ("error out"=w46:errorcluster)  [unwired: 10 in]
  n95 = while "Create an OCR session and read the character set file.\nSet paramaters from Vision Assistant Step." {
    shift-right: [w300] -> w41
    shift-left: _ -> [w299]
    tunnel: w46 -> [w302]
    tunnel: w43 -> [w298]
    tunnel: path "C:/Users/Bob Dabalina/Documents/Labview/Poker Hand2/Viewsonic1.abc" ("File Path") -> [w297]
    tunnel: [w296] -> w42
    stop <- FALSE continue-if-true
    n96 = First Call?() -> (First Call?: T/F=w301:bool)
    n97 = case shown="True" w301 {
      tunnel: w297 -> [_ w309]
      tunnel: w302 -> [w304 w313]
      tunnel: [w305 w311] -> w300
      tunnel: [w304 w310] -> w296
      tunnel: w298 -> [_ w306]
      tunnel: w299 -> [w305 _]
      frame False {
      }
      frame True {
        w314 = 0 items=["Read All", "Read Character Set Only", "Read Properties Only"] ("Read Options")
        n98 = call <vilib>:"IVA Get Alternate Path.vi"("Path In"=w309) -> ("Path Out"=w308:path)  [unwired: 10 out]
        n99 = call "IMAQ OCR Create Session"("error in (no error)"=w313) -> ("error out"=w315:errorcluster, "IMAQ OCR Session"=w316:T5)  [unwired: 9 out]
        n100 = call "IMAQ OCR Read Character Set File"("File Path"=w308, "error in (no error)"=w315, "Read Options"=w314, "IMAQ OCR Session"=w316) -> ("error out"=w312:errorcluster, "IMAQ OCR Session (dup)"=w307:T5)  [unwired: 1 in, 5 out]
        n101 = call <vilib>:"IVA OCR - Set Parameters 2.vi"("error in (no error)"=w312, "Parameters"=w306, "IMAQ OCR Session"=w307) -> ("error out"=w310:errorcluster, "IMAQ OCR Session Out"=w311:T5)  [unwired: 7 in]
      }
    }
  }
  n102 = Unbundle By Name(w43) -> ("# Lines Expected"=w39:u32, "Orientation"=w40:u32)
  n103 = call "IMAQ OCR Read Text 4"("IMAQ OCR Session"=w41, "ROI Descriptor"=w44, "Image"=w26, "Number of Lines Requested"=w39, "error in (no error)"=w42, "Orientation"=w40) -> ("Read String"=w5:string, "error out"=w38:errorcluster)  [unwired: 8 out]
  "String (Player9 OCR/OCV 4)" <- w5
  n104 = Build Array (concatenate)(w6, w5) -> (w4:string[])
  n105 = call <vilib>:"IVA Clear Coordsys Errors.vi"("error in (no error)"=w38) -> ("error out"=w37:errorcluster)  [unwired: 10 in]
  n106 = while "Create an OCR session and read the character set file.\nSet paramaters from Vision Assistant Step." {
    shift-right: [w321] -> w32
    shift-left: _ -> [w320]
    tunnel: w37 -> [w323]
    tunnel: w34 -> [w319]
    tunnel: path "C:/Users/Bob Dabalina/Documents/Labview/Poker Hand2/Viewsonic1.abc" ("File Path") -> [w318]
    tunnel: [w317] -> w33
    stop <- FALSE continue-if-true
    n107 = First Call?() -> (First Call?: T/F=w322:bool)
    n108 = case shown="True" w322 {
      tunnel: w318 -> [_ w330]
      tunnel: w323 -> [w325 w334]
      tunnel: [w326 w332] -> w321
      tunnel: [w325 w331] -> w317
      tunnel: w319 -> [_ w327]
      tunnel: w320 -> [w326 _]
      frame False {
      }
      frame True {
        w335 = 0 items=["Read All", "Read Character Set Only", "Read Properties Only"] ("Read Options")
        n109 = call <vilib>:"IVA Get Alternate Path.vi"("Path In"=w330) -> ("Path Out"=w329:path)  [unwired: 10 out]
        n110 = call "IMAQ OCR Create Session"("error in (no error)"=w334) -> ("error out"=w336:errorcluster, "IMAQ OCR Session"=w337:T5)  [unwired: 9 out]
        n111 = call "IMAQ OCR Read Character Set File"("File Path"=w329, "error in (no error)"=w336, "Read Options"=w335, "IMAQ OCR Session"=w337) -> ("error out"=w333:errorcluster, "IMAQ OCR Session (dup)"=w328:T5)  [unwired: 1 in, 5 out]
        n112 = call <vilib>:"IVA OCR - Set Parameters 2.vi"("error in (no error)"=w333, "Parameters"=w327, "IMAQ OCR Session"=w328) -> ("error out"=w331:errorcluster, "IMAQ OCR Session Out"=w332:T5)  [unwired: 7 in]
      }
    }
  }
  n113 = Unbundle By Name(w34) -> ("# Lines Expected"=w30:u32, "Orientation"=w31:u32)
  n114 = call "IMAQ OCR Read Text 4"("IMAQ OCR Session"=w32, "ROI Descriptor"=w35, "Image"=w26, "Number of Lines Requested"=w30, "error in (no error)"=w33, "Orientation"=w31) -> ("Read String"=w3:string, "error out"=w29:errorcluster)  [unwired: 8 out]
  "String ( Player10 OCR/OCV 4)" <- w3
  n115 = call <vilib>:"IVA Clear Coordsys Errors.vi"("error in (no error)"=w29) -> ("error out"=w28:errorcluster)  [unwired: 10 in]
  n116 = Build Array (concatenate)(w4, w3) -> (→"Player Names":string[])
  n117 = property on="Image Out" class="ImageControl"(error in=w28, "Palette:Palette Type"=w25) -> (error out=→"error out":errorcluster)  [unwired: 1 in, 1 out]
